vi "Edge Detect Block (SubVI).vi"(0 "Data In":u8, 7 "In Valid?":bool) -> (4 "Data Out":u8, 6 "Out Valid?":bool, 8 "X Start":u16, 10 "Y Start":u16)   [LabVIEW 2015]
uses:
  <vilib>/rvi/DataTransferAndStorage/Container/Common/niFpgaContainerGetUniqueNameForEmu.vi
  <vilib>/rvi/DataTransferAndStorage/Container/Common/niFpgaContainerSetEmuInfo.vi
  <vilib>/rvi/eio/common/nirviEmuReportErrorAndStop.vi
  <vilib>/rvi/Emulation/niFpgaEmulationIsFPGAContextNoSignature.vi
  <vilib>/rvi/Emulation/niFpgaSctlEmulationGetInTimedLoop.vi
  <vilib>/rvi/errors/niFpgaSetErrorForExecOnDevCompSimple.vi
  <vilib>/rvi/FIFO/Fifo_Resource/nirvififoEmulationSetSize.vi
  <vilib>/rvi/FIFO/Fifo_Resource/nirviFifoEmulationQueueMgr.vi
  <instcachedir>/0/nirviFifoEmulationQueueMgr_E5CAEC123FF24DC58D834DCA3CDAA9B5.lvgen/nirviFifoEmulationQueueMgr_E5CAEC123FF24DC58D834DCA3CDAA9B5_001.vi
  <vilib>/Utility/error.llb/Clear Errors.vi
  <vilib>/rvi/FIFO/Fifo_Resource/nirvififoEmulationCreateLock.vi
  <vilib>/rvi/Emulation/niFpgaProcessEmulError.vi
  <vilib>/rvi/FIFO/Fifo_Resource/nirvififoEmulationObtainLock.vi
  <vilib>/rvi/FIFO/Fifo_Resource/nirvififoEmulationReleaseLock.vi
  <vilib>/rvi/occurrence/nirviWaitOnOccurrenceBase.vi
  <vilib>/rvi/errors/nirviReportUnexpectedCaseInternalError.vi
  <vilib>/rvi/errors/nirviReportUnexpectedCaseInternalError (U32).vi
  <vilib>/rvi/FIFO/Fifo_Resource/nirvififoEmulationDetermineInputValidOut.vi
  <vilib>/rvi/LocalResourceManager/LocalResourceManager.xnode
  <vilib>/rvi/DataTransferAndStorage/Container/XNode/niFpgaContainer.xnode
  <vilib>/rvi/FIFO/Fifo_Resource/nirvififoEmulationRead.vi
  <vilib>/rvi/FIFO/Fifo_Resource/nirvififoEmulationWrite.vi
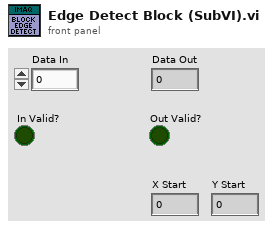
[diagram p1: front panel]
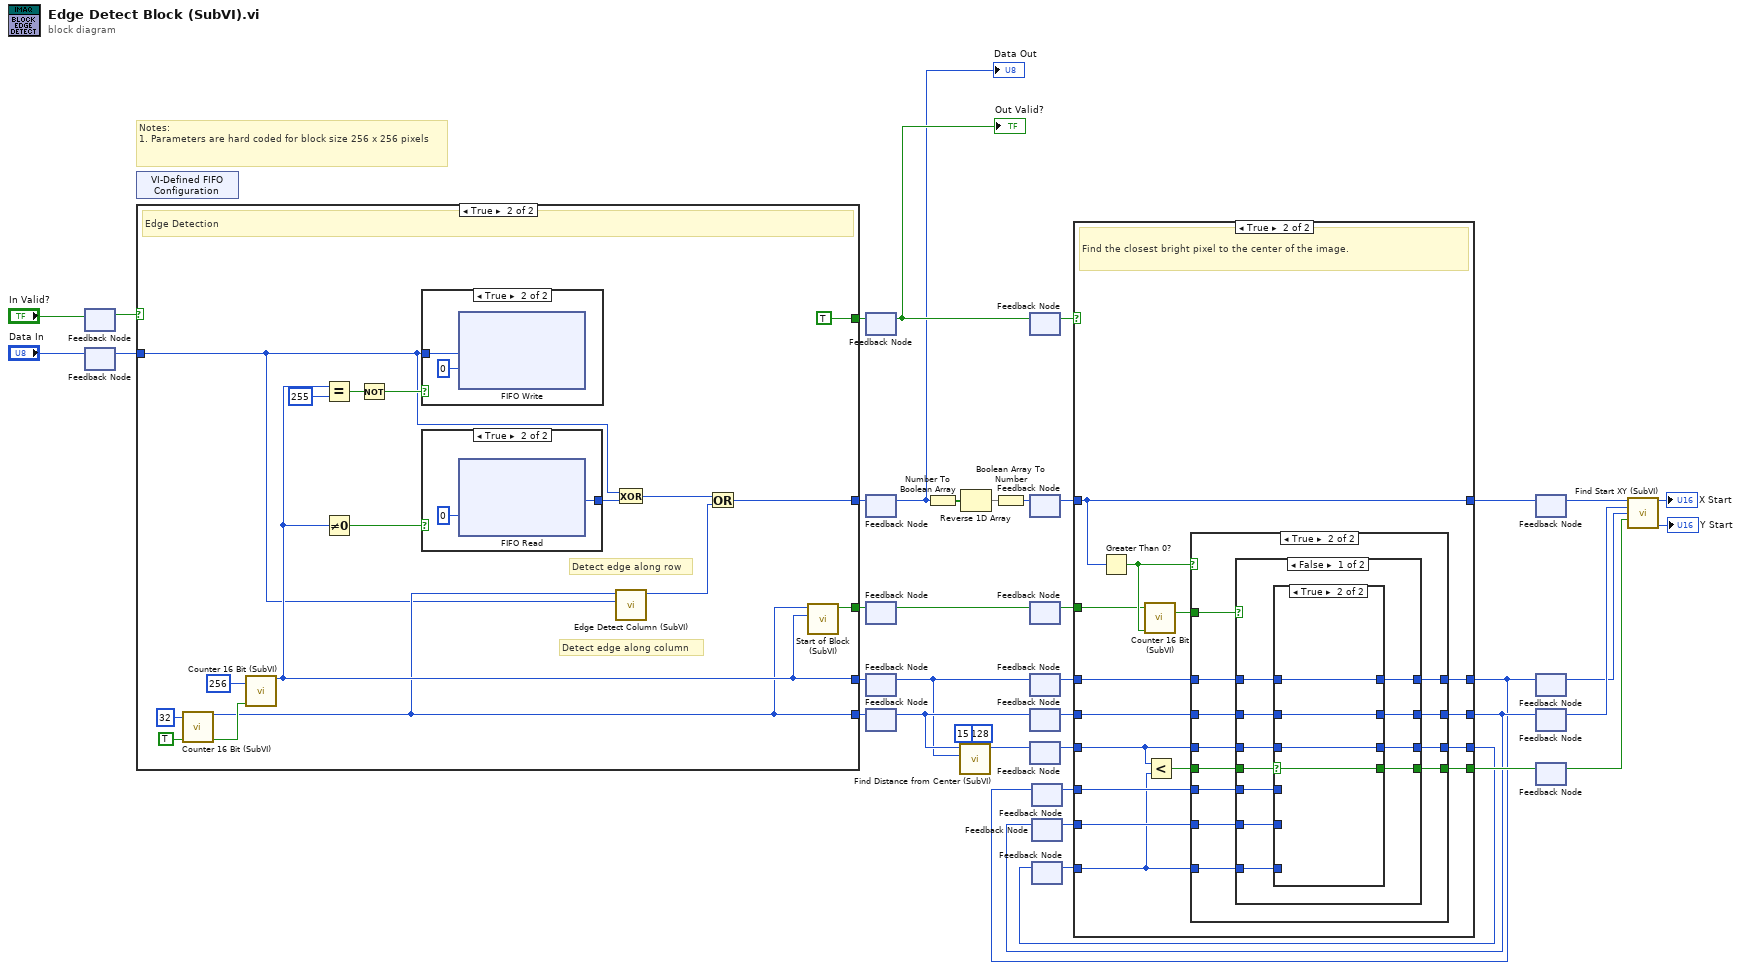
[diagram p0: block diagram]
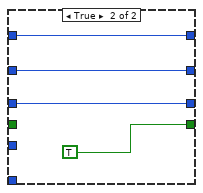
[diagram p8: hidden frame]
diagram:
  # "Notes:\n1. Parameters are hard coded for block size 256 x 256 pixels"
  n1 = feedback-in #1("In Valid?") -> ()
  n2 = feedback #1() -> (w27:bool)  [unwired: 1 in]
  n3 = feedback-in #2("Data In") -> ()
  n4 = feedback #2() -> (w5:u8)  [unwired: 1 in]
  n5 = xnode "VI-Defined FIFO Configuration"() -> ()  [unwired: 1 out]
  n6 = case shown="True" w27 {
    tunnel: w5 -> [_ w42]
    tunnel: [_ w43] -> w38
    tunnel: [_ w47] -> w37
    tunnel: [_ w41] -> w36
    tunnel: [_ TRUE ("Enable")] -> w28
    tunnel: [_ w46] -> w21
    frame False {
    }
    frame True {
      # "Detect edge along row"
      # "Detect edge along column"
      # "Edge Detection"
      n7 = call "Counter 16 Bit (SubVI).vi"("Max. Count"=u16 32, "Enable"=TRUE) -> ("Count"=w43:u16, "Count End?"=w56:bool)  [unwired: 11 in, 1 out]
      n8 = call "Counter 16 Bit (SubVI).vi"("Max. Count"=u16 256 ("Image Height"), "Enable"=w56) -> ("Count"=w47:u16)  [unwired: 11 in, 2 out]
      n9 = Equal?(x=w47, y=u16 255) -> (x = y?=w51:bool)
      n10 = Not Equal To 0?(x=w47) -> (x != 0?=w52:bool)
      n11 = Not(x=w51) -> (.not. x?=w50:bool)
      n12 = case shown="True" w50 {
        tunnel: w42 -> [_ w60]
        frame False {
        }
        frame True {
          n13 = xnode ("FIFO Write")("Element"=w60, "Timeout"=0) -> ()  [unwired: 1 in, 2 out]
        }
      }
      n14 = case shown="True" w52 {
        tunnel: [_ w58] -> w48
        frame False {
        }
        frame True {
          n15 = xnode ("FIFO Read")("Timeout"=0) -> ("Element"=w58:u8)  [unwired: 1 in, 2 out]
        }
      }
      n16 = Exclusive Or(1:w48, 2:w42) -> (0:w44:u8)
      n17 = call "Edge Detect Column (SubVI).vi"("Pixel In"=w42, "Column #"=w43) -> ("Pixel Out"=w45:u8)  [unwired: 9 in]
      n18 = Or(x=w44, y=w45) -> (x .or. y?=w41:u8)
      n19 = call "Start of Block (SubVI).vi"("Row #"=w47, "Col #"=w43) -> ("Start?"=w46:bool)  [unwired: 9 in]
    }
  }
  n20 = feedback-in #3(w28) -> ()
  n21 = feedback #3() -> (w29:bool)  [unwired: 1 in]
  "Out Valid?" <- w29
  n22 = feedback-in #4(w36) -> ()
  n23 = feedback #4() -> (w2:u8)  [unwired: 1 in]
  "Data Out" <- w2
  n24 = feedback-in #5(w21) -> ()
  n25 = feedback #5() -> (w20:bool)  [unwired: 1 in]
  n26 = feedback-in #6(w37) -> ()
  n27 = feedback #6() -> (w25:u16)  [unwired: 1 in]
  n28 = feedback-in #7(w38) -> ()
  n29 = feedback #7() -> (w26:u16)  [unwired: 1 in]
  n30 = Number To Boolean Array(number=w2) -> (Boolean array=w3:bool[])
  n31 = call "Find Distance from Center (SubVI).vi"("Y Center"=i16 128, "X Center"=i16 15, "Y"=w25, "X"=w26) -> ("Distance from Center"=w22:i16)  [unwired: 7 in]
  n32 = Reverse 1D Array(array=w3) -> (reversed array=w4:bool[])
  n33 = Boolean Array To Number(Boolean array=w4) -> (number=w1:u8)
  n34 = feedback-in #8(w29) -> ()
  n35 = feedback #8() -> (w19:bool)  [unwired: 1 in]
  n36 = feedback-in #9(w1) -> ()
  n37 = feedback #9() -> (w18:u8)  [unwired: 1 in]
  n38 = feedback-in #10(w20) -> ()
  n39 = feedback #10() -> (w15:bool)  [unwired: 1 in]
  n40 = feedback-in #11(w25) -> ()
  n41 = feedback #11() -> (w16:u16)  [unwired: 1 in]
  n42 = feedback-in #12(w26) -> ()
  n43 = feedback #12() -> (w14:u16)  [unwired: 1 in]
  n44 = feedback-in #13(w22) -> ()
  n45 = feedback #13() -> (w17:i16)  [unwired: 1 in]
  n46 = feedback #14() -> (w33:u16)  [unwired: 1 in]
  n47 = feedback #15() -> (w32:u16)  [unwired: 1 in]
  n48 = feedback #16() -> (w12:i16)  [unwired: 1 in]
  n49 = case shown="True" w19 {
    tunnel: w16 -> [_ w74]
    tunnel: w14 -> [_ w73]
    tunnel: w18 -> [_ w79]
    tunnel: [_ w79] -> w35
    tunnel: [w64 w75] -> w30
    tunnel: [w63 w76] -> w31
    tunnel: [_ w77] -> w34
    tunnel: w33 -> [w64 w72]
    tunnel: w32 -> [w63 w71]
    tunnel: w17 -> [_ w66]
    tunnel: w15 -> [_ w69]
    tunnel: [w62 w68] -> w13
    tunnel: w12 -> [w62 w67]
    frame False {
    }
    frame True {
      # "Find the closest bright pixel to the center of the image."
      n50 = Greater Than 0?(x=w79) -> (x > 0?=w70:bool)
      n51 = call "Counter 16 Bit (SubVI).vi"("RESET"=w69, "Enable"=w70) -> ("Count Begin?"=w78:bool)  [unwired: 11 in, 2 out]
      n52 = Less?(x=w66, y=w67) -> (x < y?=w65:bool)
      n53 = case shown="True" w70 {
        tunnel: w78 -> [_ w94]
        tunnel: [_ w93] -> w77
        tunnel: [w81 w92] -> w76
        tunnel: [w82 w91] -> w75
        tunnel: w74 -> [_ w90]
        tunnel: w73 -> [_ w89]
        tunnel: w72 -> [w82 w88]
        tunnel: w71 -> [w81 w87]
        tunnel: w66 -> [_ w86]
        tunnel: [w80 w85] -> w68
        tunnel: w67 -> [w80 w84]
        tunnel: w65 -> [_ w83]
        frame False {
        }
        frame True {
          n54 = case shown="False" w94 {
            tunnel: [w95 TRUE] -> w93
            tunnel: w90 -> [w105 w115]
            tunnel: w89 -> [w104 w116]
            tunnel: [w102 w116] -> w92
            tunnel: [w103 w115] -> w91
            tunnel: w88 -> [w101 _]
            tunnel: w87 -> [w100 _]
            tunnel: w86 -> [w99 w113]
            tunnel: [w98 w113] -> w85
            tunnel: w84 -> [w97 _]
            tunnel: w83 -> [w96 _]
            frame False {
              n55 = case shown="True" w96 {
                selector: w96 -> [_ w109]
                tunnel: w105 -> [_ w112]
                tunnel: w104 -> [_ w111]
                tunnel: [w108 w112] -> w103
                tunnel: [w107 w111] -> w102
                tunnel: w101 -> [w108 _]
                tunnel: w100 -> [w107 _]
                tunnel: w99 -> [_ w110]
                tunnel: [w106 w110] -> w98
                tunnel: w97 -> [w106 _]
                tunnel: [_ w109] -> w95
                frame False {
                }
                frame True {
                }
              }
            }
            frame True {
            }
          }
        }
      }
    }
  }
  n56 = feedback-in #14(w30) -> ()
  n57 = feedback-in #15(w31) -> ()
  n58 = feedback-in #16(w13) -> ()
  n59 = feedback #17() -> (w9:u8)  [unwired: 1 in]
  n60 = feedback-in #17(w35) -> ()
  n61 = feedback #18() -> (w7:u16)  [unwired: 1 in]
  n62 = feedback-in #18(w30) -> ()
  n63 = feedback #19() -> (w8:u16)  [unwired: 1 in]
  n64 = feedback-in #19(w31) -> ()
  n65 = feedback #20() -> (w6:bool)  [unwired: 1 in]
  n66 = feedback-in #20(w34) -> ()
  n67 = call "Find Start XY (SubVI).vi"("Data In"=w9, "xStart In"=w8, "yStart In"=w7, "Fnd?"=w6) -> ("xStart"=→"X Start":u16, "yStart"=→"Y Start":u16)  [unwired: 10 in]
